vi "Part 2.vi"(11 "Input":string) -> (3 "Output":i64)   [LabVIEW 2021]
uses:
  <userlib>/_OpenG.lib/string/string.llb/Convert EOLs (String)__ogtk.vi
panel:
  out "In Range?":bool
  in  "Test":i32=2
  # "902 = too high\n883 = too low\n893 = too low\n\nNot\n898\n899\n900\n\nCORRECT\n894"
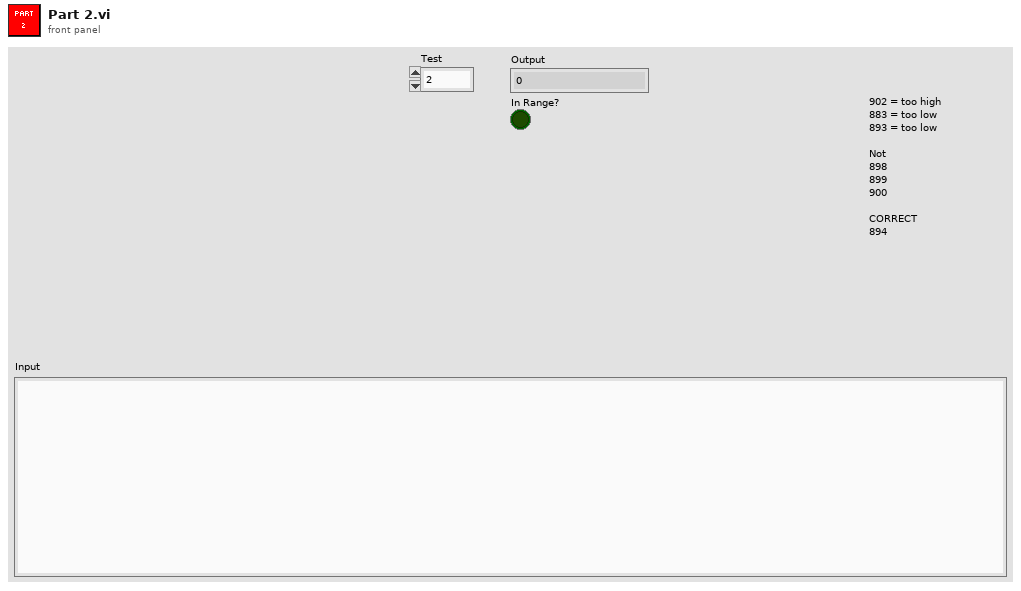
[diagram p1: front panel]
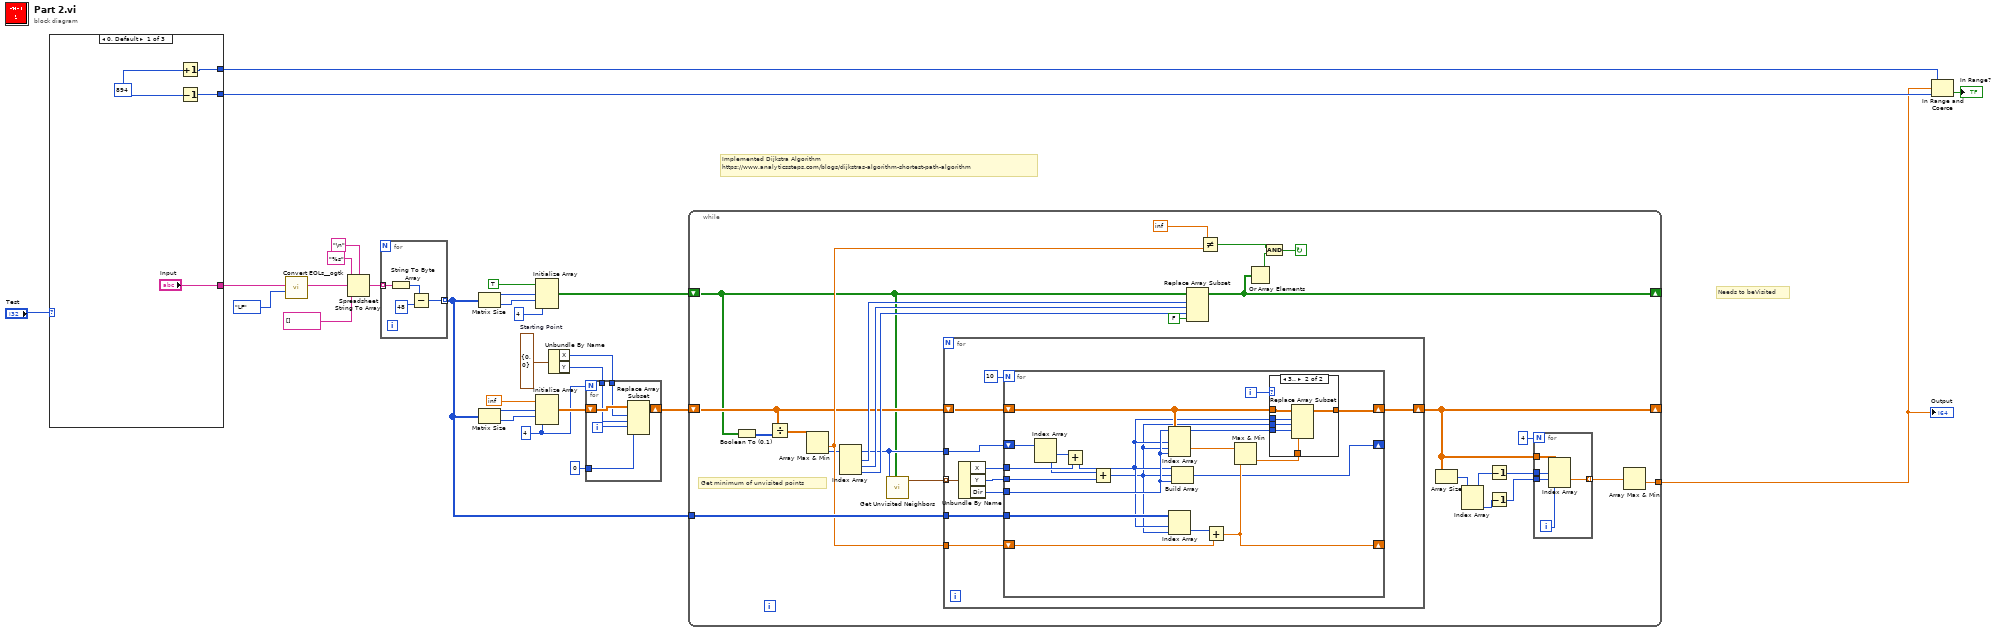
[diagram p0: block diagram]
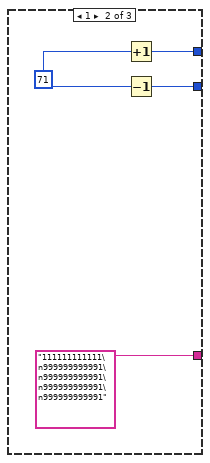
[diagram p3: hidden frame]
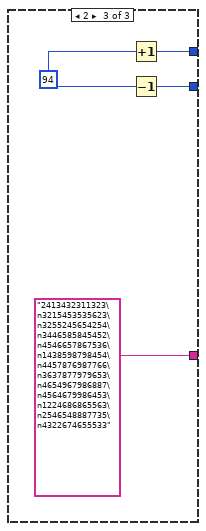
[diagram p4: hidden frame]
diagram:
  w10 = 4
  w15 = cluster{"X":i32, "Y":i32} {"X"=0, "Y"=0}  # Starting Point
  # "Implemented Dijkstra Algorithm\nhttps://www.analyticssteps.com/blogs/dijkstras-algorithm-shortest-path-algorithm"
  # "Needs to beVisited"
  n1 = case shown="0, Default" "Test" {
    tunnel: ["Input" "111111111111\n999999999991\n999999999991\n999999999991\n999999999991" "2413432311323\n3215453535623\n3255245654254\n3446585845452\n4546657867536\n1438598798454\n4457876987766\n3637877979653\n4654967986887\n4564679986453\n1224686865563\n2546548887735\n4322674655533"] -> w5
    tunnel: [w30 w34 w38] -> w3
    tunnel: [w29 w33 w37] -> w2
    frame 0, Default {
      w31 = 894
      n2 = Increment(x=w31) -> (x+1=w30:i32)
      n3 = Decrement(x=w31) -> (x-1=w29:i32)
    }
    frame 1 {
      w35 = 71
      n4 = Increment(x=w35) -> (x+1=w34:i32)
      n5 = Decrement(x=w35) -> (x-1=w33:i32)
    }
    frame 2 {
      w39 = 94
      n6 = Increment(x=w39) -> (x+1=w38:i32)
      n7 = Decrement(x=w39) -> (x-1=w37:i32)
    }
  }
  n8 = call-poly <userlib>:"Convert EOLs__ogtk.vi"("Convert to:"=enum16{"CR", "LF", "CRLF"}."LF", "String in"=w5) -> ("String out"=w25:string)  [unwired: 9 in]
  n9 = Spreadsheet String To Array(delimiter (Tab)="\n", format string="%s", spreadsheet string=w25, array type (2D Dbl)=string[] []) -> (array=w23:string[])
  n10 = for {
    tunnel: w23 -> [w44] mode=indexing
    tunnel: [w41] -> w9 mode=indexing
    n11 = String To Byte Array(string=w44) -> (unsigned byte array=w43:u8[])
    n12 = Subtract(x=w43, y=u8 48) -> (x-y=w41:u8[])
  }
  n13 = Matrix Size(0:w9) -> (1:w22:i32, 2:w11:i32)
  n14 = Matrix Size(0:w9) -> (1:w18:i32, 2:w12:i32)
  n15 = Initialize Array(TRUE, w22, w11, 4) -> (w20:bool[][][])
  n16 = Initialize Array(inf, w18, w12, w10) -> (w19:dbl[][][])
  n17 = Unbundle By Name(w15) -> ("X"=w13:i32, "Y"=w14:i32)
  n18 = for {
    N: w10 -> [_]
    tunnel: w14 -> [w48]
    tunnel: w13 -> [w47]
    shift-right: [w49] -> w16
    shift-left: w19 -> [w50]
    tunnel: u8 0 -> [w45]
    i -> [w46]
    n19 = Replace Array Subset(array=w50, new element=w45, index (dim 0)=w47, index (dim 1)=w48, index (dim 2)=w46) -> (w49:dbl[][][])
  }
  n20 = while {
    shift-right: [w72] -> _
    shift-left: w20 -> [w61]
    shift-right: [w53] -> _
    shift-left: w16 -> [w62]
    tunnel: w9 -> [w75]
    tunnel: [w52] -> w1
    stop <- w66 continue-if-true
    # "Get minimum of unvisited points"
    n21 = Boolean To (0,1)(Boolean=w61) -> (0, 1=w70:i16[][][])
    n22 = Divide(x=w62, y=w70) -> (x/y=w69:dbl[][][])
    n23 = Array Max & Min(array=w69) -> (min value=w64:dbl, min index (indices)=w63:i32[])  [unwired: 2 out]
    n24 = Index Array(array=w63) -> (element #1=w74:i32, element #2=w73:i32, element #3=w68:i32)  [unwired: 3 in]
    n25 = call "Get Unvisited Neighbors.vi"("Unvisited"=w61, "Current Point"=w63) -> ("Unvisited Neighbors"=w71:cluster{"X":i32, "Y":i32, "Dir":i32}[])  [unwired: 9 in]
    n26 = for {
      tunnel: w75 -> [w91]
      tunnel: w71 -> [w85] mode=indexing
      tunnel: w64 -> [w88]
      shift-right: [w90] -> w53
      shift-left: w62 -> [w89]
      tunnel: w63 -> [w86]
      n27 = Unbundle By Name(w85) -> ("X"=w84:i32, "Y"=w83:i32, "Dir"=w82:i32)
      n28 = for {
        N: 10 -> [_]
        shift-right: [w107] -> w90
        shift-left: w89 -> [w108]
        tunnel: w91 -> [w106]
        shift-right: [w105] -> _
        shift-left: w88 -> [w109]
        shift-right: [w102] -> _
        shift-left: w86 -> [w104]
        tunnel: w84 -> [w100]
        tunnel: w83 -> [w97]
        tunnel: w82 -> [w103]
        i -> [w93]
        n29 = Index Array(array=w104) -> (element #1=w101:i32, element #2=w98:i32)  [unwired: 2 in]
        n30 = Add(x=w101, y=w100) -> (x+y=w99:i32)
        n31 = Add(x=w98, y=w97) -> (x+y=w92:i32)
        n32 = Index Array(array=w108, index (dim 0)=w99, index (dim 1)=w92, index (dim 2)=w103) -> (element=w96:dbl)
        n33 = Index Array(array=w106, index (row)=w99, index (col)=w92) -> (element=w95:u8)
        n34 = Build Array(w99, w92, w103) -> (w102:i32[])
        n35 = Add(x=w95, y=w109) -> (x+y=w105:dbl)
        n36 = Max & Min(x=w96, y=w105) -> (min(x,y)=w94:dbl)  [unwired: 1 out]
        n37 = case shown="3.." w93 {
          tunnel: w108 -> [w110 w116]
          tunnel: [w110 w115] -> w107
          tunnel: w103 -> [_ w114]
          tunnel: w99 -> [_ w113]
          tunnel: w92 -> [_ w112]
          tunnel: w94 -> [_ w111]
          frame ..2 {
          }
          frame 3.. {
            n38 = Replace Array Subset(array=w116, new element=w111, index (dim 0)=w113, index (dim 1)=w112, index (dim 2)=w114) -> (w115:dbl[][][])
          }
        }
      }
    }
    n39 = Replace Array Subset(array=w61, new element=FALSE, index (dim 0)=w74, index (dim 1)=w73, index (dim 2)=w68) -> (w72:bool[][][])
    n40 = Not Equal?(x=inf, y=w64) -> (x != y?=w51:bool)
    n41 = Or Array Elements(Boolean array=w72) -> (logical OR=w67:bool)
    n42 = And(x=w51, y=w67) -> (x .and. y?=w66:bool)
    n43 = Array Size(array=w53) -> (size(s)=w58:i32[])
    n44 = Index Array(array=w58) -> (element #1=w59:i32, element #2=w60:i32)  [unwired: 2 in]
    n45 = Decrement(x=w59) -> (x-1=w55:i32)
    n46 = Decrement(x=w60) -> (x-1=w57:i32)
    n47 = for {
      N: 4 -> [_]
      tunnel: w55 -> [w81]
      tunnel: w53 -> [w80]
      tunnel: [w79] -> w56 mode=indexing
      tunnel: w57 -> [w78]
      i -> [w77]
      n48 = Index Array(array=w80, index (dim 0)=w81, index (dim 1)=w78, index (dim 2)=w77) -> (element=w79:dbl)
    }
    n49 = Array Max & Min(array=w56) -> (min value=w52:dbl)  [unwired: 3 out]
  }
  "Output" <- w1
  n50 = In Range and Coerce(upper limit=w3, x=w1, lower limit=w2) -> (In Range?=→"In Range?":bool)  [unwired: 1 out]
